vi "PI String Array to Comma List.vi"(10 "No Spaces?":bool, 11 "Array":string[](array[string])) -> (3 "String":string)   [LabVIEW 2011]
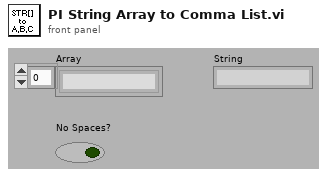
[diagram p1: front panel]
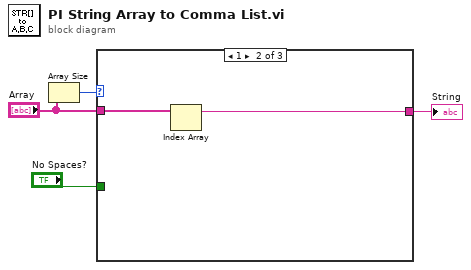
[diagram p0: block diagram]
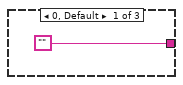
[diagram p2: hidden frame]
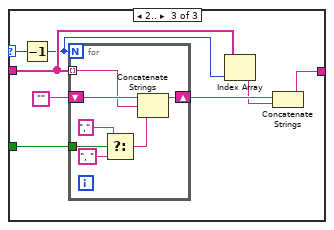
[diagram p3: hidden frame]
diagram:
  n1 = Array Size(array="Array") -> (size(s)=w2:i32)
  n2 = case shown="1" w2 {
    selector: w2 -> [_ _ w15]
    tunnel: ["" w6 w9] -> w3
    tunnel: "Array" -> [_ w7 w13]
    tunnel: "No Spaces?" -> [_ _ w8]
    frame 0, Default {
    }
    frame 1 {
      n3 = Index Array(array=w7) -> (element=w6:string)  [unwired: 1 in]
    }
    frame 2.. {
      n4 = Decrement(x=w15) -> (x-1=w12:i32)
      n5 = for {
        N: w12 -> [_]
        tunnel: w13 -> [w21] mode=indexing
        shift-right: [w20] -> w11
        shift-left: "" -> [w22]
        tunnel: w8 -> [w18]
        n6 = Select(t=",", s=w18, f=", ") -> (s? t:f=w16:string)
        n7 = Concatenate Strings(w22, w21, w16) -> (w20:string)
      }
      n8 = Index Array(array=w13, index=w12) -> (element=w10:string)
      n9 = Concatenate Strings(w11, w10) -> (w9:string)
    }
  }
  "String" <- w3
